vi "Destroy.vi"(8 "error in":errorcluster, 11 "Logger in":refnum<class "Logger.lvclass">) -> (0 "error out":errorcluster, 3 "Logger out":refnum<class "Logger.lvclass">)   [LabVIEW 2020, in "hse-logger.lvlib" / "Logger.lvclass"]
doc: "Closes all handlers and removes them from the logger.\n\n____\nHAMPEL SOFTWARE ENGINEERING v2.0.6 (2021-04-15 11:38)"
uses:
  Logger.lvclass
  Handler/Handler.lvclass
  Logger.lvclass/Logger.ctl
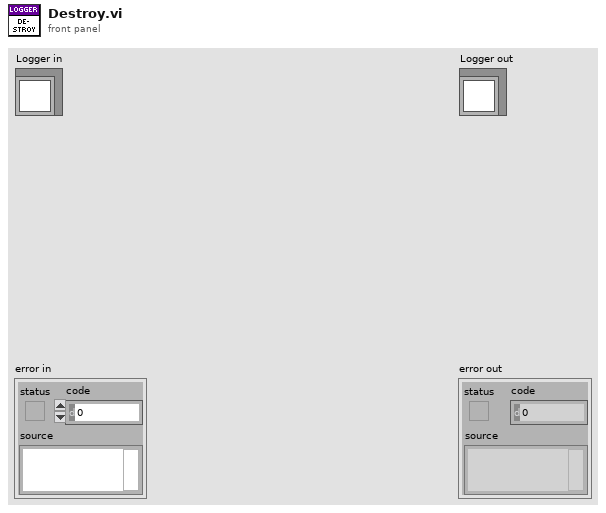
[diagram p1: front panel]
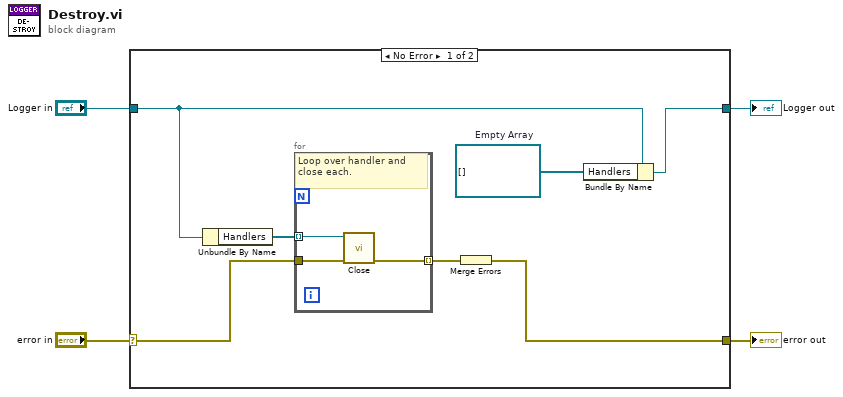
[diagram p0: block diagram]
diagram:
  n1 = case shown="No Error" "error in" {
    selector: "error in" -> [w10 w16]
    tunnel: [w5 w16] -> w3
    tunnel: [w7 w15] -> w1
    tunnel: "Logger in" -> [w8 w15]
    frame No Error {
      w6 = refnum<class "Handler.lvclass">[] []  # Empty Array
      n2 = Unbundle By Name(w8) -> ("Handlers"=w11:refnum<class "Handler.lvclass">[])
      n3 = for {
        tunnel: w11 -> [w14] mode=indexing
        tunnel: w10 -> [w13]
        tunnel: [w12] -> w9 mode=indexing
        # "Loop over handler and close each."
        n4 = call-dynamic "Close.vi"("error in"=w13, "Handler in"=w14) -> ("error out"=w12:errorcluster)  [unwired: 8 in, 1 out]
      }
      n5 = Merge Errors(w9) -> (w5:errorcluster)
      n6 = Bundle By Name(cluster=w8, "Handlers"=w6) -> (w7:refnum<class "Logger.lvclass">)
    }
    frame Error {
    }
  }
  "error out" <- w3
  "Logger out" <- w1
